vi "Write Return Device IED_Status Msg.vi"(10 "Return Device IED_Status Msg":refnum<class "Return Device IED_Status Msg.lvclass">, 11 "Manual Control in":refnum<class "Manual Control.lvclass">) -> (3 "Manual Control out":refnum<class "Manual Control.lvclass">)   [LabVIEW 2016]
uses:
  Manual Control.lvclass
  C:/Users/Administrator/Desktop/LabVIEW EMS/Optimization/Generic Optimization Actor/Generic Optimization/Generic Optimization.lvclass
  C:/Users/Administrator/Desktop/LabVIEW EMS/SCADA Sub Abstract Actor/SCADA Sub Abstract/SCADA Sub Abstract.lvclass
  C:/Users/Administrator/Desktop/LabVIEW EMS/EMS Generic Actor/EMS Generic/EMS Generic.lvclass
  C:/Program Files (x86)/National Instruments/LabVIEW 2016/vi.lib/ActorFramework/Actor/Actor.lvclass
  Manual Control Messages/Return Device IED_Status Msg/Return Device IED_Status Msg.lvclass
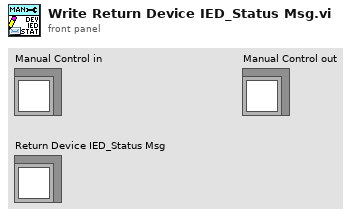
[diagram p1: front panel]
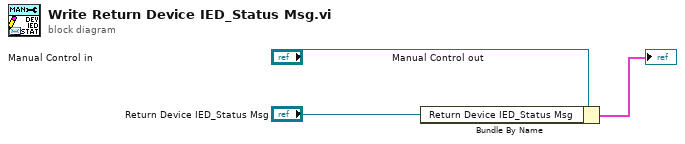
[diagram p0: block diagram]
diagram:
  n1 = Bundle By Name(cluster="Manual Control in", "Return Device IED_Status Msg"="Return Device IED_Status Msg") -> (→"Manual Control out":cluster{})
